vi "ods.vi"(2 "error in (no error)":errorcluster, 3 "str":string) -> (0 "error out":errorcluster)   [LabVIEW 2015]
uses:
  kernel32.dll
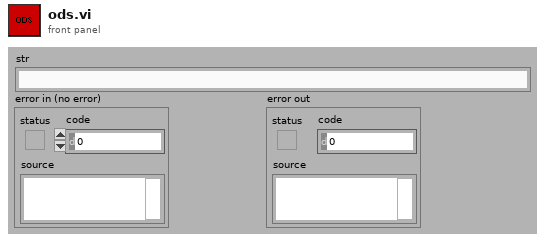
[diagram p1: front panel]
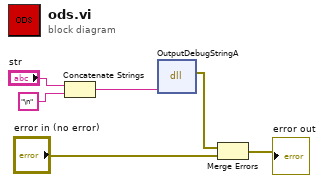
[diagram p0: block diagram]
diagram:
  n1 = Concatenate Strings("str", "\n") -> (w4:string)
  n2 = dll-call lib="kernel32.dll" fn="OutputDebugStringA"("str"=w4) -> (error out=w1:errorcluster)  [unwired: 4 in, 2 out]
  n3 = Merge Errors(w1, "error in (no error)") -> (→"error out":errorcluster)
